vi "BlinkM GetRGB.vi"(8 "Error In":errorcluster, 10 "Address":u8, 11 "ChipKit Resource":T1={"COM Port"="", "Board Type"=enum."ChipKit uC32", "Connection Type"=enum."USB / Serial", "Baud Rate (115200)"=15, "Bytes Per Packet (15)"=15}) -> (0 "Error Out":errorcluster, 2 "Color":u32(colorbox), 3 "ChipKit Resource":T1={"COM Port"="", "Board Type"=enum."ChipKit uC32", "Connection Type"=enum."USB / Serial", "Baud Rate (115200)"=15, "Bytes Per Packet (15)"=15})   [LabVIEW 2011, in "LabVIEW Interface for ChipKit.lvlib"]
doc: "Get the current RGB color of the specified BlinkM."
uses:
  LabVIEW Interface for ChipKit.lvlib
  Private/Type Defs/Chipkit Resource.ctl
  Private/Type Defs/Board Type.ctl
  Private/Type Defs/Connection Type.ctl
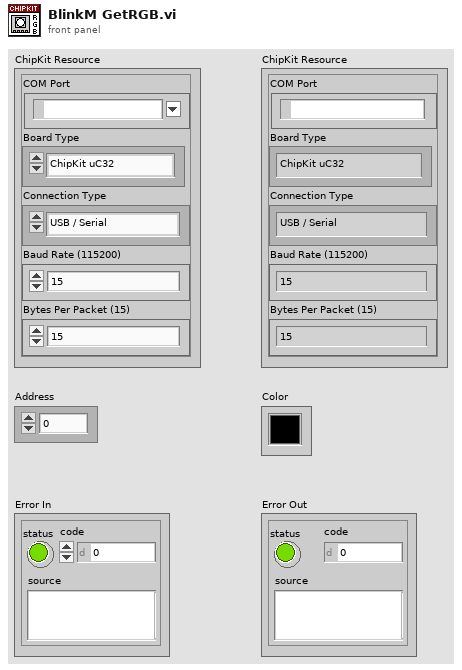
[diagram p1: front panel]
types:
  T1 = typedef "LabVIEW Interface for ChipKit.lvlib/Chipkit Resource.ctl" = cluster{"COM Port":refnum<visa-resource-name>, "Board Type":T2, "Connection Type":T3, "Baud Rate (115200)":u32, "Bytes Per Packet (15)":u32}
  T2 = typedef "LabVIEW Interface for ChipKit.lvlib/Board Type.ctl" = enum16{"ChipKit uC32", "ChipKit Uno32", "ChipKit Max32"}
  T3 = typedef "LabVIEW Interface for ChipKit.lvlib/Connection Type.ctl" = enum8{"USB / Serial", "XBEE", "BlueSmirf (Bluetooth)"}
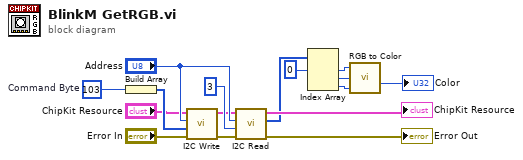
[diagram p0: block diagram]
diagram:
  w15 = u8 103  # Command Byte
  n1 = Build Array(w15) -> (w14:u8[])
  n2 = call "I2C Write.vi"("Error In"="Error In", "I2C Data"=w14, "Address (0)"="Address", "ChipKit Resource"="ChipKit Resource") -> ("Error Out"=w13:errorcluster, "ChipKit Resource"=w4:T1)  [unwired: 6 in]
  n3 = call "I2C Read.vi"("Error In"=w13, "Bytes To Read"=u8 3, "Address (0)"="Address", "ChipKit Resource"=w4) -> ("Error Out"=→"Error Out":errorcluster, "I2C Data"=w2:u8[], "ChipKit Resource"=→"ChipKit Resource":T1)  [unwired: 5 in]
  n4 = Index Array(array=w2, index #1=0 ("index")) -> (element #1=w8:u8, element #2=w7:u8, element #3=w6:u8)  [unwired: 2 in]
  n5 = call <vilib>:"RGB to Color.vi"("B"=w6, "G"=w7, "R"=w8) -> ("Color"=→"Color":u32)
